vi "TankDrive.vi"(4 "AccelRate":dbl, 5 "Cutoff":dbl=0.15 format="%#_13g", 6 "LoopTime":dbl, 7 "DriveAction":T9, 8 "error in (no error)":errorcluster, 9 "RightDesired":dbl, 10 "LeftDesired":dbl, 11 "RobotDriveDevRef":T1={"DevStatus"={"status"=FALSE, "code"=0, "source"=""}, "Motors[]"=[], "Square Inputs"=FALSE, "Max Output"=1.0, "Isochronous"=FALSE}) -> (0 "error out":errorcluster)   [LabVIEW 2013]
doc: "Straight drive True locks both motor desired values to the left joystick.\nHalf drive True divides desired values by 2 to allow more fine controls. This does not half the accel rate."
uses:
  TankDriveAction.ctl
  <vilib>/Rock Robotics/WPI/RobotDrive/WPI_RobotDriveDevRef.ctl
  <vilib>/Rock Robotics/WPI/MotorControl/WPI_MotorControlDeviceRef.ctl
  <vilib>/Rock Robotics/SystemInterfaces/Typedef/FPGA_TypedefDigitalModule.ctl
  <vilib>/Rock Robotics/SystemInterfaces/DIO/FPGA_DIOPWMChannel.ctl
  <vilib>/Rock Robotics/WPI/PWM/WPI_PWMDeadband.ctl
  <vilib>/Rock Robotics/WPI/CAN/Jaguar/SubVIs/WPI_CANJaguar_ControlMode.ctl
  <vilib>/Rock Robotics/WPI/PWM/WPI_PWMTransform_ConPane.ctl
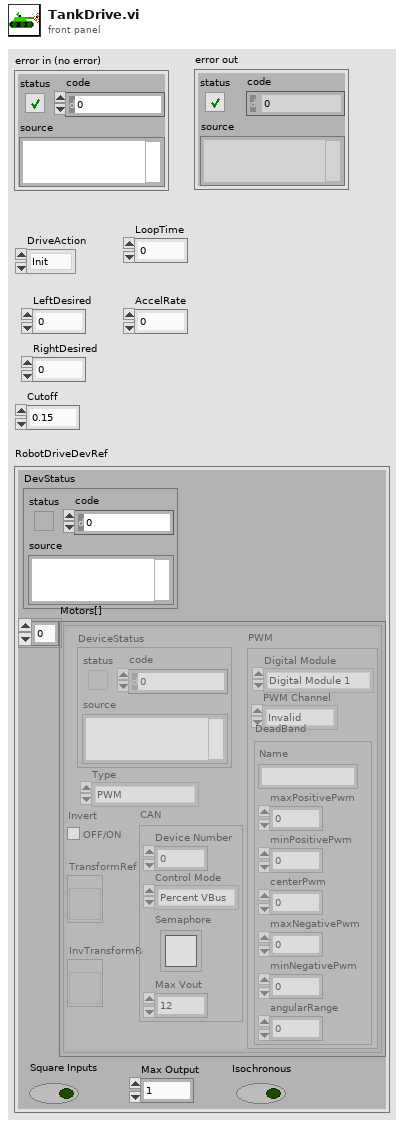
[diagram p1: front panel]
types:
  T1 = typedef "WPI_RobotDriveDevRef.ctl" = cluster{"DevStatus":errorcluster, "Motors[]":T2[], "Square Inputs":bool, "Max Output":dbl, "Isochronous":bool}
  T2 = typedef "WPI_MotorControlDeviceRef.ctl" = cluster{"DeviceStatus":errorcluster, "Type":enum16{"PWM", "CAN"}, "PWM":cluster{"Digital Module":T3, "PWM Channel":T4, "DeadBand":T5}, "CAN":cluster{"Device Number":u8, "Control Mode":T6, "Semaphore":T7, "Max Vout":dbl}, "Invert":bool, "TransformRef":T8, "InvTransformRef":T8}
  T3 = typedef "FPGA_TypedefDigitalModule.ctl" = enum16{"Digital Module 1", "Digital Module 2"}
  T4 = typedef "FPGA_DIOPWMChannel.ctl" = enum8{"PWM 1", "PWM 2", "PWM 3", "PWM 4", "PWM 5", "PWM 6", "PWM 7", "PWM 8", "PWM 9", "PWM 10", "Invalid"}
  T5 = typedef "WPI_PWMDeadband.ctl" = cluster{"Name":string, "maxPositivePwm":i32, "minPositivePwm":i32, "centerPwm":i32, "maxNegativePwm":i32, "minNegativePwm":i32, "angularRange":u16}
  T6 = typedef "WPI_CANJaguar_ControlMode.ctl" = enum8{"Percent VBus", "Current", "Speed", "Position", "Voltage"}
  T7 = typedef "Semaphore RefNum" = refnum<k1>
  T8 = typedef "WPI_PWMTransform_ConPane.ctl" = refnum<vi>
  T9 = typedef "TankDriveAction.ctl" = enum16{"Init", "LinearDrive", "SetValue", "Disable"}
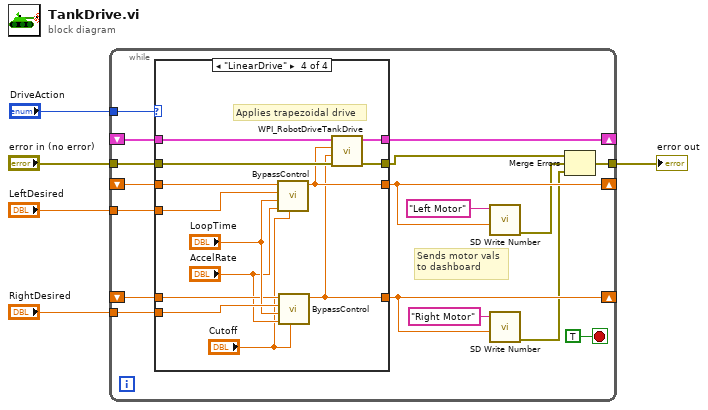
[diagram p0: block diagram]
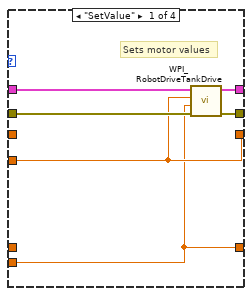
[diagram p2: hidden frame]
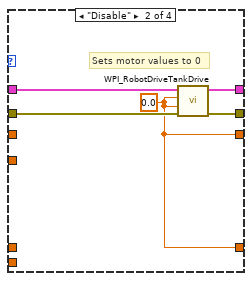
[diagram p3: hidden frame]
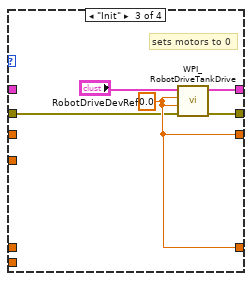
[diagram p4: hidden frame]
diagram:
  n1 = while {
    shift-right: [w22] -> _
    shift-left: _ -> [w20]
    tunnel: "error in (no error)" -> [w17]
    tunnel: "DriveAction" -> [w16]
    tunnel: "LeftDesired" -> [w15]
    tunnel: "RightDesired" -> [w14]
    shift-right: [w12] -> _
    shift-left: _ -> [w13]
    shift-right: [w11] -> _
    shift-left: _ -> [w10]
    tunnel: [w9] -> w1
    stop <- TRUE stop-if-true
    # "Sends motor vals\nto dashboard"
    n2 = case shown="\"LinearDrive\"" w16 {
      tunnel: [w23 w32 w36 w44] -> w22
      tunnel: w20 -> [w24 w33 _ w43]
      tunnel: w17 -> [w28 w31 w34 w50]
      tunnel: [w27 w30 w38 w51] -> w8
      tunnel: [w26 w29 w37 w47] -> w12
      tunnel: [w25 w29 w37 w46] -> w11
      tunnel: w15 -> [w26 _ _ w49]
      tunnel: w14 -> [w25 _ _ w48]
      tunnel: w13 -> [_ _ _ w42]
      tunnel: w10 -> [_ _ _ w41]
      frame "SetValue" {
        # "Sets motor values"
        n3 = call <vilib>:"WPI_RobotDriveTankDrive.vi"("error in (no error)"=w28, "Right axis value"=w25, "Left axis value"=w26, "RobotDriveDevRef"=w24) -> ("error out"=w27:errorcluster, "RobotDriveDevRef"=w23:T1)  [unwired: 5 in, 1 out]
      }
      frame "Disable" {
        w29 = 0.0
        # "Sets motor values to 0"
        n4 = call <vilib>:"WPI_RobotDriveTankDrive.vi"("error in (no error)"=w31, "Right axis value"=w29, "Left axis value"=w29, "RobotDriveDevRef"=w33) -> ("error out"=w30:errorcluster, "RobotDriveDevRef"=w32:T1)  [unwired: 5 in, 1 out]
      }
      frame "Init" {
        w37 = 0.0
        # "sets motors to 0"
        n5 = call <vilib>:"WPI_RobotDriveTankDrive.vi"("error in (no error)"=w34, "Right axis value"=w37, "Left axis value"=w37, "RobotDriveDevRef"="RobotDriveDevRef") -> ("error out"=w38:errorcluster, "RobotDriveDevRef"=w36:T1)  [unwired: 5 in, 1 out]
      }
      frame "LinearDrive" {
        # "Applies trapezoidal drive"
        n6 = call "BypassControl.vi"("Cutoff"="Cutoff", "AccelRate"="AccelRate", "LoopTime"="LoopTime", "DesiredInput"=w49, "CurrentInput"=w42) -> ("SetMotor"=w47:dbl)  [unwired: 6 in]
        n7 = call "BypassControl.vi"("Cutoff"="Cutoff", "AccelRate"="AccelRate", "LoopTime"="LoopTime", "DesiredInput"=w48, "CurrentInput"=w41) -> ("SetMotor"=w46:dbl)  [unwired: 6 in]
        n8 = call <vilib>:"WPI_RobotDriveTankDrive.vi"("error in (no error)"=w50, "Right axis value"=w46, "Left axis value"=w47, "RobotDriveDevRef"=w43) -> ("error out"=w51:errorcluster, "RobotDriveDevRef"=w44:T1)  [unwired: 5 in, 1 out]
      }
    }
    n9 = call <vilib>:"SD Write Number.vi"("Numeric"=w12, "Name"="Left Motor") -> ("error out"=w7:errorcluster)  [unwired: 8 in, 1 out]
    n10 = call <vilib>:"SD Write Number.vi"("Numeric"=w11, "Name"="Right Motor") -> ("error out"=w6:errorcluster)  [unwired: 8 in, 1 out]
    n11 = Merge Errors(w8, w7, w6) -> (w9:errorcluster)
  }
  "error out" <- w1
